vi "6-7素材.vi"() -> ()   [LabVIEW 2018]
uses:
  <vilib>/measure/maspectr.llb/FFT Spectrum (Mag-Phase) for 1 Chan.vi
  <vilib>/measure/maspectr.llb/FFT Spectrum (Mag-Phase) for N Chan.vi
  <vilib>/measure/NI_MABase.lvlib
  <vilib>/measure/NI_MAPro.lvlib
panel:
  in  "选项卡控件":enum32{"调制", "滤波"}(tab)
  out "混频后频谱图":cluster{"f0":dbl, "df":dbl, "magnitude":dbl[]}(graph)
  out "两个信号频域图":cluster{"f0":dbl, "df":dbl, "magnitude":dbl[]}[](graph)
  out "混频时域图":waveform(dbl)(graph)
  out "两个信号时域图":waveform(dbl)[](graph)
  in  "调制系数":dbl(slide) min=0.0 max=1.0 scale=0.0..1.0
  in  "信号频率":dbl(slide)=10.0 min=0.0 max=10.0 scale=0.0..10.0
  in  "signal type":T1(ring) caption="信号类型"
  in  "载波频率":dbl(slide)=40.0 min=40.0 max=100.0 scale=40.0..100.0
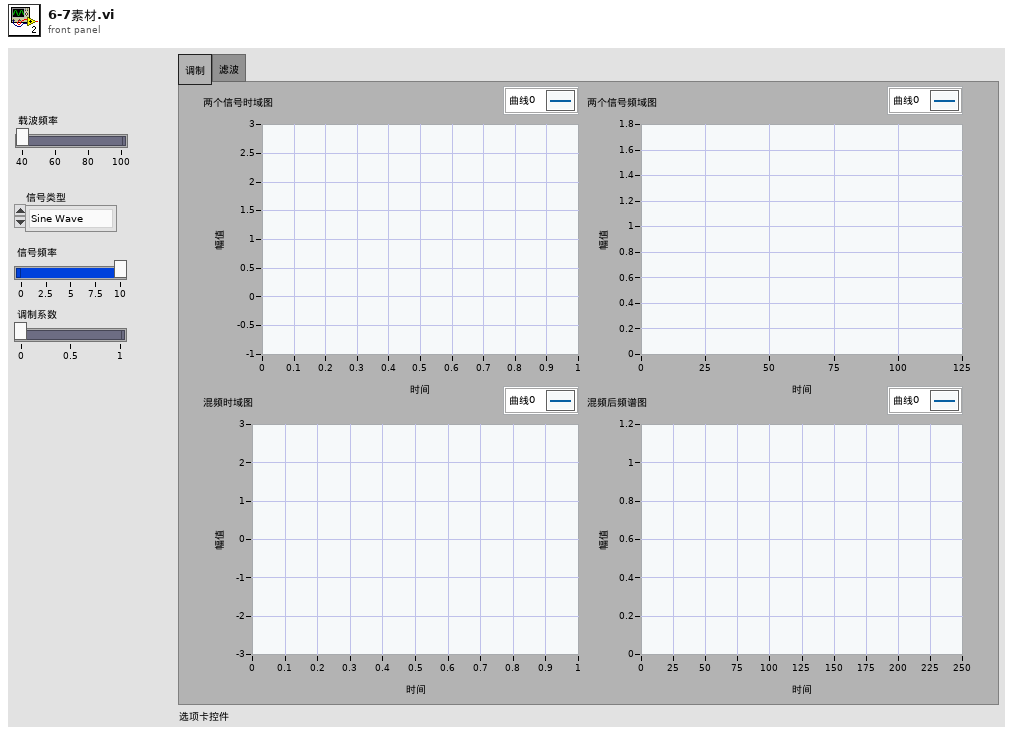
[diagram p1: front panel]
types:
  T1 = enum16{"Sine Wave", "Triangle Wave", "Square Wave", "Sawtooth Wave"}
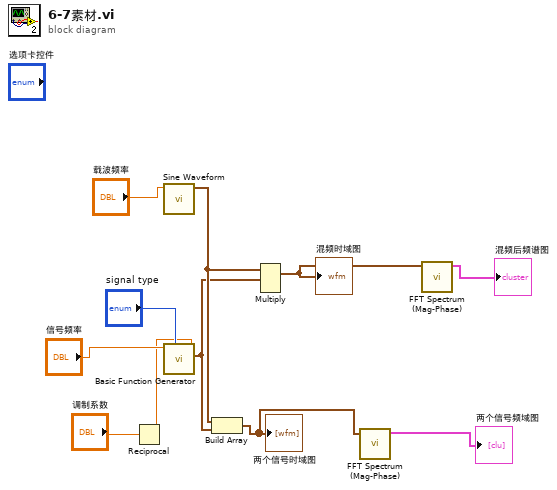
[diagram p0: block diagram]
diagram:
  n1 = Reciprocal(x="调制系数") -> (1/x=w7:dbl)
  n2 = call <vilib>:"Sine Waveform.vi"("frequency"="载波频率") -> ("signal out"=w6:waveform(dbl))  [unwired: 9 in, 1 out]
  n3 = call <vilib>:"Basic Function Generator.vi"("offset"=w7, "signal type"="signal type", "frequency"="信号频率") -> ("signal out"=w5:waveform(dbl))  [unwired: 6 in, 2 out]
  n4 = Build Array(w6, w5) -> (w3:waveform(dbl)[])
  "两个信号时域图" <- w3
  n5 = Multiply(1:w5, 2:w6) -> (0:w4:waveform(dbl))  [unwired: 1 in, 1 out]
  "混频时域图" <- w4
  n6 = call-poly <vilib>:"FFT Spectrum (Mag-Phase).vi"("time signals"=w3) -> ("magnitudes"=→"两个信号频域图":cluster{"f0":dbl, "df":dbl, "magnitude":dbl[]}[])  [unwired: 6 in, 4 out]
  n7 = call-poly <vilib>:"FFT Spectrum (Mag-Phase).vi"("time signal"=w4) -> ("magnitude"=→"混频后频谱图":cluster{"f0":dbl, "df":dbl, "magnitude":dbl[]})  [unwired: 6 in, 4 out]
